vi "To String.vi"(8 "error in (no error)":errorcluster, 11 "Formatter Config in":refnum<class "Formatter Config.lvclass">) -> (0 "error out":errorcluster, 2 "data":string, 3 "Formatter Config out":refnum<class "Formatter Config.lvclass">)   [LabVIEW 2015, in "Formatter Config.lvclass"]
uses:
  Formatter Config.lvclass
  Formatter Config.lvclass/Formatter Config.ctl
  <vilib>/NI/Configuration Framework/serializable configuration/NISE_CEF_serializable configuration.lvclass
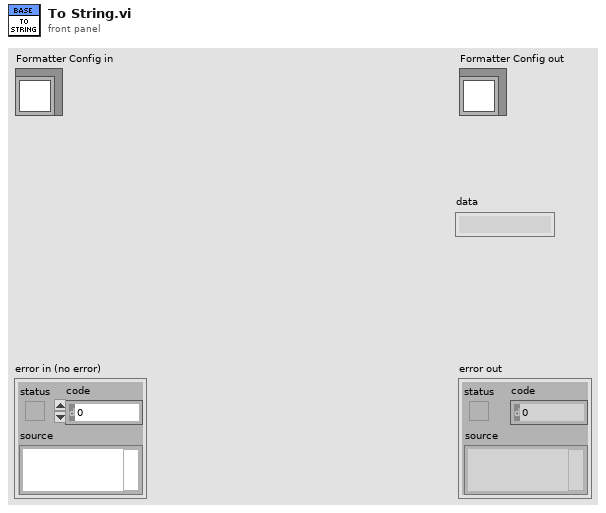
[diagram p1: front panel]
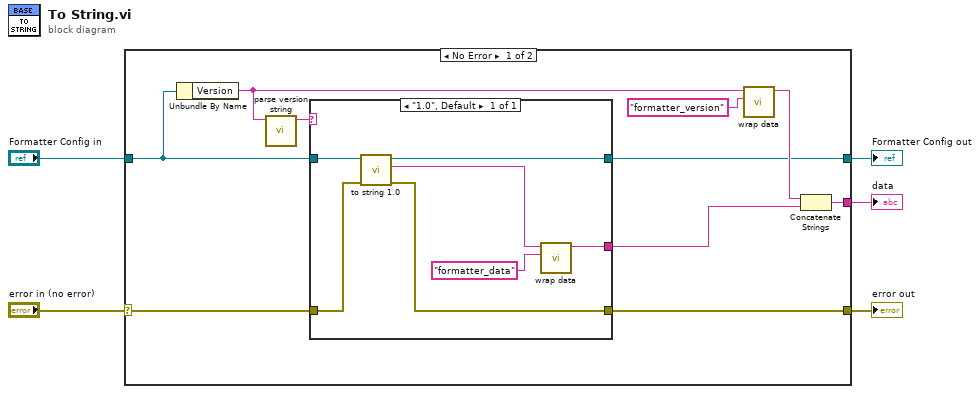
[diagram p0: block diagram]
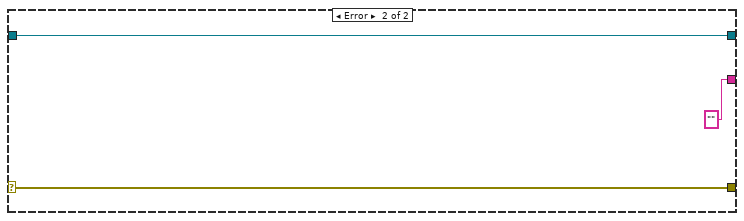
[diagram p2: hidden frame]
diagram:
  n1 = case shown="No Error" "error in (no error)" {
    selector: "error in (no error)" -> [w6 w25]
    tunnel: [w7 w25] -> w4
    tunnel: [w8 w24] -> w2
    tunnel: "Formatter Config in" -> [w9 w24]
    tunnel: [w12 ""] -> w1
    frame No Error {
      n2 = Unbundle By Name(w9) -> ("Version"=w11:string)
      n3 = call <vilib>:"parse version string.vi"("full version"=w11) -> ("major.minor version"=w10:string)  [unwired: 7 in, 3 out]
      n4 = case shown="\"1.0\", Default" w10 {
        tunnel: [w21] -> w13
        tunnel: w9 -> [w20]
        tunnel: [w19] -> w8
        tunnel: [w17] -> w7
        tunnel: w6 -> [w16]
        frame "1.0", Default {
          n5 = call-dynamic "to string 1.0.vi"("error in (no error)"=w16, "Formatter Config in"=w20) -> ("error out"=w17:errorcluster, "data"=w18:string, "Formatter Config out"=w19:refnum<class "Formatter Config.lvclass">)  [unwired: 7 in]
          n6 = call <vilib>:"wrap data.vi"("identifier"="formatter_data", "data to wrap"=w18) -> ("wrapped data"=w21:string)  [unwired: 9 in]
        }
      }
      n7 = call <vilib>:"wrap data.vi"("identifier"="formatter_version", "data to wrap"=w11) -> ("wrapped data"=w14:string)  [unwired: 9 in]
      n8 = Concatenate Strings(w14, w13) -> (w12:string)
    }
    frame Error {
    }
  }
  "error out" <- w4
  "Formatter Config out" <- w2
  "data" <- w1
